vi "gugudan Client.vi"() -> ()   [LabVIEW 2014]
uses:
  <vilib>/Utility/sysdir.llb/System Directory Type.ctl
  <vilib>/regexp/Match Regular Expression.xnode
  <vilib>/FTP/NI_FTP.lvlib
panel:
  out "ip address":string=" ip address\r\n   서브넷 마스크 . . . . . . . : 255.255.255.0\r\n   기본 게이트웨이 . . . . . . : 192.168.0.1\r\n\r\n터널 어댑터 isatap.{E2E91750-802C-47E4-94E7-F6C5BD44A78B}:\r\n\r\n   미디어 상태 . . . . . . . . : 미디어 연결 끊김\r\n   연결별 DNS 접미사. . . . : \r\n\r\n터널 어댑터 로컬 영역 연결* 2:\r\n\r\n   연결별 DNS 접미사. . . . : \r\n   IPv6 주소 . . . . . . . . . : 2001:0:682f:9980:3c40:17a9:3f57:fff6\r\n   링크-로컬 IPv6 주소 . . . . : fe80::3c40:17a9:3f57:fff6%12\r\n   기본 게이트웨이 . . . . . . : ::\r\n"
  in  "제한해제":bool
  out "TIME":string="현재날자,시간"
  out "배열":string[][](array[string])
  out "email":string
  out "abs(x)":i32
  out "문자열":string
  out "스페이스바3 2":string
  out "W":string
  out "1":string
  out "2":string
  out "3":string
  # "서비스를 이용해 주셔 감사합니다."
  # "서비스 종료를 위해서는 관리자 암호를 입력 해야 종료가 가능합니다."
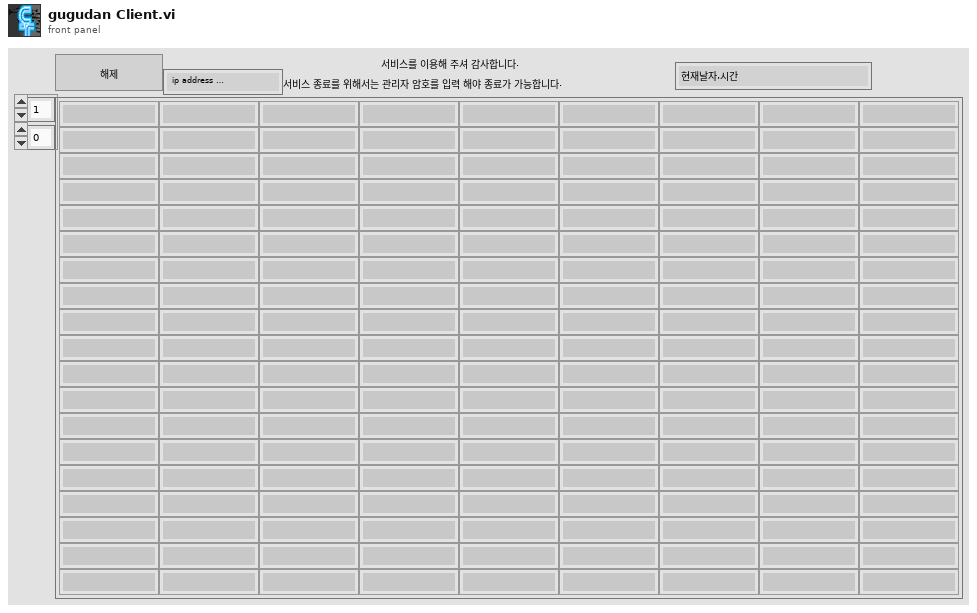
[diagram p1: front panel]
types:
  T1 = enum16{"open", "replace", "create", "open or create", "replace or create", "replace or create with confirmation"}
  T2 = typedef "System Directory Type.ctl" = i32
  T3 = typedef "NI_FTP.lvlib/FTP Session.ctl" = refnum<k5>
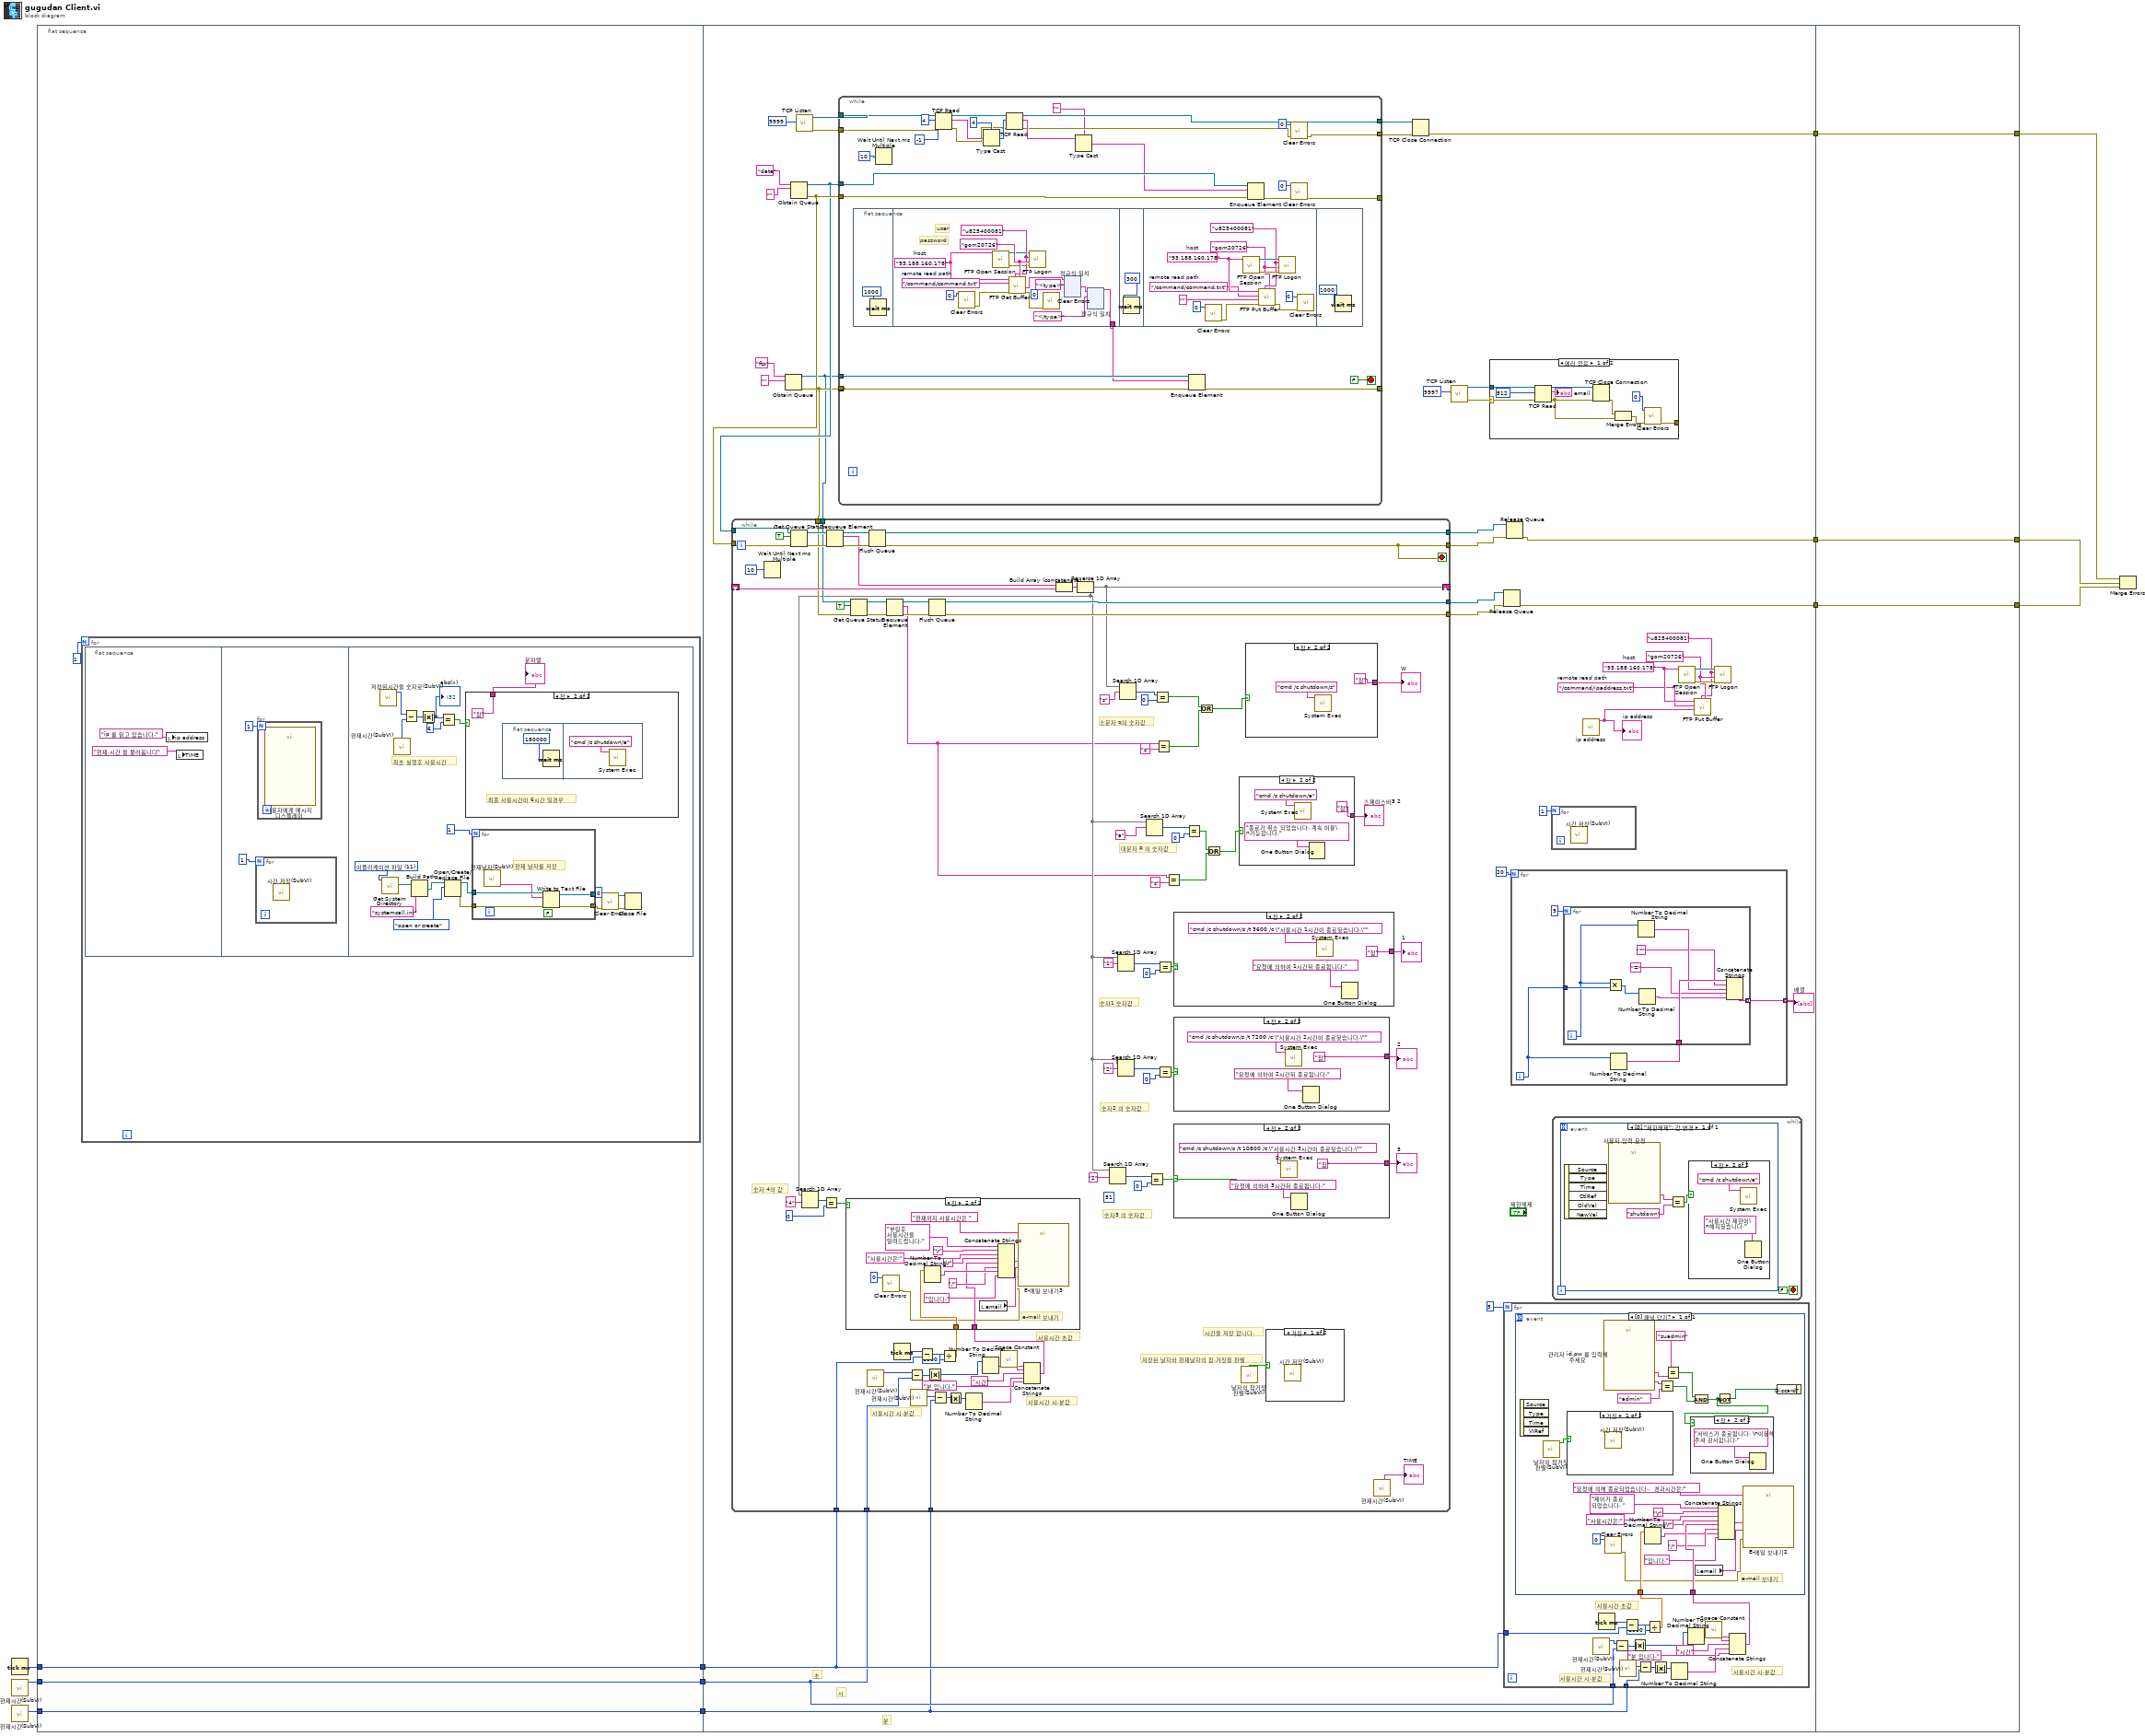
[diagram p0: block diagram]
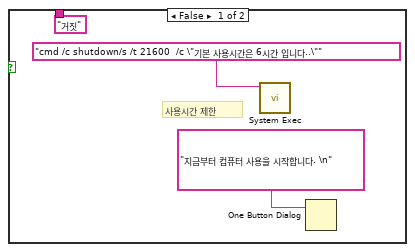
[diagram p2: hidden frame]
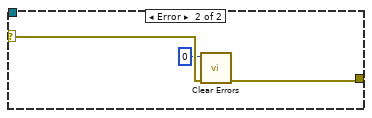
[diagram p4: hidden frame]
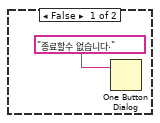
[diagram p6: hidden frame]
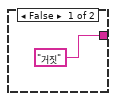
[diagram p9: hidden frame]
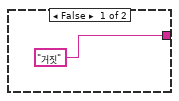
[diagram p10: hidden frame]
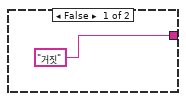
[diagram p11: hidden frame]
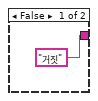
[diagram p12: hidden frame]
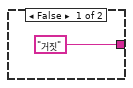
[diagram p13: hidden frame]
diagram:
  n1 = Tick Count (ms)() -> (millisecond timer value=w6:u32)
  n2 = call "현재시간(SubVI).vi"() -> ("시"=w5:i32)  [unwired: 3 in, 8 out]
  n3 = call "현재시간(SubVI).vi"() -> ("분"=w4:i32)  [unwired: 3 in, 8 out]
  n4 = flat-sequence {
    tunnel: [w15] -> w7
    tunnel: w6 -> [w15]
    tunnel: w5 -> [w14]
    tunnel: w4 -> [w13]
    tunnel: [w14] -> w3
    tunnel: [w13] -> w2
    tunnel: [w77] -> w12
    tunnel: [w73] -> w11
    tunnel: [w76] -> w10
    tunnel: w7 -> [w71]
    tunnel: w3 -> [w70]
    tunnel: w2 -> [w69]
    tunnel: w12 -> [w562]
    tunnel: w11 -> [w561]
    tunnel: w10 -> [w560]
    tunnel: [w562] -> w9
    tunnel: [w561] -> w8
    tunnel: [w560] -> w1
    frame #0 {
      n5 = for {
        N: 1 -> [_]
        n6 = flat-sequence {
          frame #0 {
            n7 = local write "ip address"("ip 를 읽고 있습니다.") -> ()
            n8 = local write "TIME"("현재,시간 을 불러옵니다") -> ()
          }
          frame #1 {
            n9 = for {
              N: 1 -> [_]
              n10 = call "시간 저장(SubVI).vi"() -> ()  [unwired: 12 in]
            }
            n11 = for {
              N: 1 -> [_]
              n12 = call "사용자에게 메시지 디스플레이"() -> ()  [unwired: 10 in, 2 out]
            }
          }
          frame #2 {
            w23 = T2 11 items=["사용자 홈"=0, "사용자 데스크탑"=1, "사용자 문서"=2, "사용자 어플리케이션 데이터"=3, "사용자 환경"=4, "사용자 임시"=5, "퍼블릭 문서"=6, "퍼블릭 어플리케이션 데이터"=7, "퍼블릭 환경"=8, "퍼블릭 캐시"=13, "시스템 코어 라이브러리"=9, "시스템 설치된 라이브러리"=10, "어플리케이션 파일"=11, "부팅 볼륨 루트"=12] ("system directory type")
            # "최초 실행후 사용시간"
            n13 = call "저장된시간을 숫자로(SubVI).vi"() -> ("저장된 문자를 숫자로"=w33:i32)  [unwired: 11 in]
            n14 = call <vilib>:"Get System Directory.vi"("system directory type"=w23) -> ("system directory"=w28:path)  [unwired: 10 in]
            n15 = call "현재시간(SubVI).vi"() -> ("시"=w34:i32)  [unwired: 3 in, 8 out]
            n16 = Subtract(x=w33, y=w34) -> (x-y=w35:i32)
            n17 = Build Path(base path=w28, name or relative path="systemcall.ini" ("이름 또는 상대 경로")) -> (appended path=w26:path)
            n18 = Absolute Value(x=w35) -> (abs(x)=w37:i32)
            "abs(x)" <- w37
            n19 = Equal?(x=w37, y=6) -> (x = y?=w39:bool)
            n20 = Open/Create/Replace File(file path (use dialog)=w26, operation (0:open)=T1."open or create" ("동작(0:open)")) -> (refnum out=w24:refnum<file>, error out=w25:errorcluster)  [unwired: 4 in, 1 out]
            n21 = case shown="참" w39 {
              tunnel: ["거짓" "참"] -> w36
              frame False {
                # "사용시간 제한"
                n22 = call <vilib>:"System Exec.vi"("command line"="cmd /c shutdown/s /t 21600  /c \"기본 사용시간은 6시간 입니다..\"" ("standard input")) -> ()  [unwired: 7 in, 4 out]
                n23 = One Button Dialog(message="지금부터 컴퓨터 사용을 시작합니다. \n" ("메시지")) -> ()  [unwired: 1 in, 1 out]
              }
              frame True {
                # "최종 사용시간이 6시간 일경우"
                n24 = flat-sequence {
                  frame #0 {
                    n25 = Wait (ms)(milliseconds to wait=u32 180000 ("대기 시간(ms)")) -> ()  [unwired: 1 out]
                  }
                  frame #1 {
                    n26 = call <vilib>:"System Exec.vi"("command line"="cmd /c shutdown/a" ("standard input")) -> ()  [unwired: 7 in, 4 out]
                  }
                }
              }
            }
            "문자열" <- w36
            n27 = for {
              N: 1 -> [_]
              tunnel: w25 -> [w44]
              tunnel: [w43] -> w30
              tunnel: [w42] -> w29
              tunnel: w24 -> [w41]
              (unwired) FALSE
              # "현재 날자를 저장"
              n28 = call "현재날자(SubVI).vi"() -> ("월,일 을 문자열로"=w40:string)  [unwired: 5 in, 6 out]
              n29 = Write to Text File(file (use dialog)=w41, text=w40, error in=w44) -> (refnum out=w42:refnum<file>, error out=w43:errorcluster)  [unwired: 1 in, 1 out]
            }
            n30 = call <vilib>:"Clear Errors.vi"("error in (no error)"=w30, "specific error code to clear (0: all)"=0) -> ("error out"=w31:errorcluster)  [unwired: 4 in, 1 out]
            n31 = Close File(refnum=w29, error in=w31) -> ()  [unwired: 2 out]
          }
        }
      }
    }
    frame #1 {
      w60 = "gom20726"
      w57 = "u825400081"
      w58 = "/command/ipaddress.txt"  # remote read path
      w59 = "93.188.160.178"  # host
      # "초"
      # "분"
      # "시"
      n32 = Obtain Queue(name (unnamed)="ftp" ("이름(이름없음)"), element data type="") -> (queue out=w52:refnum<queue>, error out=w53:errorcluster)  [unwired: 3 in, 1 out]
      n33 = Obtain Queue(name (unnamed)="data" ("이름(이름없음)"), element data type="") -> (queue out=w80:refnum<queue>, error out=w81:errorcluster)  [unwired: 3 in, 1 out]
      n34 = while {
        shift-right: [w175] -> _
        shift-left: _ -> [w227]
        tunnel: [w220] -> w83
        tunnel: [w219] -> w82
        tunnel: w80 -> [w226]
        tunnel: w81 -> [w225]
        tunnel: [w210] -> w79
        tunnel: [w209] -> w78
        tunnel: w52 -> [w205]
        tunnel: w53 -> [w204]
        tunnel: w71 -> [w185]
        tunnel: w70 -> [w184]
        tunnel: w69 -> [w183]
        stop <- w219 stop-if-true
        (unwired) i16 51 ("원소")
        # "숫자 4의 값"
        # "저장된 날자와 현재날자의 참,거짓을 판별"
        # "시간을 저장 합니다."
        # "사용시간 시,분값"
        # "사용시간 시,분값"
        # "사용시간 초값"
        # "대문자 R 의 숫자값"
        # "숫자3 의 숫자값"
        # "소문자 q의 숫자값"
        # "숫자1 숫자값"
        # "숫자2 의 숫자값"
        n35 = Wait Until Next ms Multiple(millisecond multiple=u32 10) -> ()  [unwired: 1 out]
        n36 = Get Queue Status(queue=w226, return elements? (F)=TRUE ("원소 반환? (거짓)"), error in (no error)=w225) -> (queue out=w224:refnum<queue>, error out=w223:errorcluster)  [unwired: 6 out]
        n37 = Dequeue Element(queue=w224, error in (no error)=w223) -> (queue out=w221:refnum<queue>, element=w218:string, error out=w222:errorcluster)  [unwired: 1 in, 1 out]
        n38 = Get Queue Status(queue=w205, return elements? (F)=TRUE ("원소 반환? (거짓)"), error in (no error)=w204) -> (queue out=w214:refnum<queue>, error out=w213:errorcluster)  [unwired: 6 out]
        n39 = call "현재시간(SubVI).vi"() -> ("시"=w187:i32)  [unwired: 3 in, 8 out]
        n40 = Flush Queue(queue=w221, error in (no error)=w222) -> (queue out=w220:refnum<queue>, error out=w219:errorcluster)  [unwired: 1 out]
        n41 = Dequeue Element(queue=w214, error in (no error)=w213) -> (queue out=w211:refnum<queue>, element=w167:string, error out=w212:errorcluster)  [unwired: 1 in, 1 out]
        n42 = Tick Count (ms)() -> (millisecond timer value=w186:u32)
        n43 = Subtract(x=w187, y=w184) -> (x-y=w189:i32)
        n44 = call "현재시간(SubVI).vi"() -> ("분"=w188:i32)  [unwired: 3 in, 8 out]
        n45 = Subtract(x=w186, y=w185) -> (x-y=w198:u32)
        n46 = Absolute Value(x=w189) -> (abs(x)=w191:i32)
        n47 = Flush Queue(queue=w211, error in (no error)=w212) -> (queue out=w209:refnum<queue>, error out=w210:errorcluster)  [unwired: 1 out]
        n48 = Subtract(x=w188, y=w183) -> (x-y=w190:i32)
        n49 = Divide(x=w198, y=u32 1000) -> (x/y=w182:dbl)
        n50 = Absolute Value(x=w190) -> (abs(x)=w192:i32)
        n51 = Number To Decimal String(number=w192) -> (decimal integer string=w194:string)  [unwired: 1 in]
        n52 = Number To Decimal String(number=w191) -> (decimal integer string=w196:string)  [unwired: 1 in]
        n53 = call <vilib>:"Space Constant.vi"() -> ("String"=w197:string)
        n54 = Concatenate Strings(w196, w197, "시간", w194, "분 입니다.") -> (w181:string)
        n55 = Build Array (concatenate)(w218, w227) -> (w216:string[])
        n56 = Reverse 1D Array(array=w216) -> (reversed array=w175:string[])
        n57 = Search 1D Array(1D array=w175, element="4") -> (index of element=w202:i32)  [unwired: 1 in]
        n58 = Equal?(x=w202, y=0) -> (x = y?=w200:bool)
        n59 = case shown="참" w200 {
          tunnel: w182 -> [_ w248]
          tunnel: w181 -> [_ w247]
          frame False {
          }
          frame True {
            # "e-mail 보내기"
            n60 = call <vilib>:"Clear Errors.vi"("specific error code to clear (0: all)"=0) -> ("error out"=w244:errorcluster)  [unwired: 5 in, 1 out]
            n61 = Number To Decimal String(number=w248) -> (decimal integer string=w256:string)  [unwired: 1 in]
            n62 = local read "email"() -> (w246:string)
            n63 = Concatenate Strings("부팅후 사용시간을 알려드립니다." ("문자열"), "\r", "사용시간은:", "\r", w247, "/", w256, "입니다.") -> (w253:string)
            n64 = call "E-메일 보내기3"("error in"=w244, "Message"=w253, "Subject"="현재까지 사용시간은 ", "Recipients"=w246) -> ()  [unwired: 7 in, 1 out]
          }
        }
        n65 = Search 1D Array(1D array=w175, element="2") -> (index of element=w232:i32)  [unwired: 1 in]
        n66 = Search 1D Array(1D array=w175, element="1" ("원소")) -> (index of element=w240:i32)  [unwired: 1 in]
        n67 = Search 1D Array(1D array=w175, element="2" ("원소")) -> (index of element=w233:i32)  [unwired: 1 in]
        n68 = Search 1D Array(1D array=w175, element="s" ("원소")) -> (index of element=w242:i32)  [unwired: 1 in]
        n69 = Search 1D Array(1D array=w175, element="a" ("원소")) -> (index of element=w207:i32)  [unwired: 1 in]
        n70 = Equal?(x=w232, y=0) -> (x = y?=w230:bool)
        n71 = Equal?(x=w242, y=0) -> (x = y?=w171:bool)
        n72 = Equal?(x=w167, y="s") -> (x = y?=w170:bool)
        n73 = Equal?(x=w240, y=0) -> (x = y?=w238:bool)
        n74 = Equal?(x=w233, y=0) -> (x = y?=w235:bool)
        n75 = Equal?(x=w167, y="s") -> (x = y?=w165:bool)
        n76 = case shown="참" w238 {
          tunnel: ["거짓" "참"] -> w239
          frame False {
          }
          frame True {
            n77 = call <vilib>:"System Exec.vi"("command line"="cmd /c shutdown/s /t 3600 /c \"사용시간 1시간이 종료됫습니다.\"" ("standard input")) -> ()  [unwired: 7 in, 4 out]
            n78 = One Button Dialog(message="요청에 의하여 1시간뒤 종료됩니다." ("메시지")) -> ()  [unwired: 1 in, 1 out]
          }
        }
        "1" <- w239
        n79 = case shown="참" w235 {
          tunnel: ["거짓" "참"] -> w234
          frame False {
          }
          frame True {
            n80 = call <vilib>:"System Exec.vi"("command line"="cmd /c shutdown/s /t 7200 /c \"사용시간 2시간이 종료됫습니다.\"" ("standard input")) -> ()  [unwired: 7 in, 4 out]
            n81 = One Button Dialog(message="요청에 의하여 2시간뒤 종료됩니다." ("메시지")) -> ()  [unwired: 1 in, 1 out]
          }
        }
        "2" <- w234
        n82 = case shown="참" w230 {
          tunnel: ["거짓" "참"] -> w217
          frame False {
          }
          frame True {
            n83 = call <vilib>:"System Exec.vi"("command line"="cmd /c shutdown/s /t 10800 /c \"사용시간 3시간이 종료됫습니다.\"" ("standard input")) -> ()  [unwired: 7 in, 4 out]
            n84 = One Button Dialog(message="요청에 의하여 3시간뒤 종료됩니다." ("메시지")) -> ()  [unwired: 1 in, 1 out]
          }
        }
        "3" <- w217
        n85 = Equal?(x=w207, y=0) -> (x = y?=w166:bool)
        n86 = Or(x=w171, y=w170) -> (x .or. y?=w169:bool)
        n87 = Or(x=w166, y=w165) -> (x .or. y?=w164:bool)
        n88 = case shown="참" w164 {
          tunnel: ["거짓" "참"] -> w206
          frame False {
          }
          frame True {
            n89 = call <vilib>:"System Exec.vi"("command line"="cmd /c shutdown/a" ("standard input")) -> ()  [unwired: 7 in, 4 out]
            n90 = One Button Dialog(message="종료가 취소 되었습니다. 계속 이용\n가능합니다." ("메시지")) -> ()  [unwired: 1 in, 1 out]
          }
        }
        "스페이스바3 2" <- w206
        n91 = call "날자의 참거짓 판별(SubVI).vi"() -> ("불리언"=w203:bool)  [unwired: 9 in, 2 out]
        n92 = case shown="참" w169 {
          tunnel: ["거짓" "참"] -> w243
          frame False {
          }
          frame True {
            n93 = call <vilib>:"System Exec.vi"("command line"="cmd /c shutdown/s" ("standard input")) -> ()  [unwired: 7 in, 4 out]
          }
        }
        "W" <- w243
        n94 = case shown="거짓" w203 {
          frame False {
            n95 = call "시간 저장(SubVI).vi"() -> ()  [unwired: 12 in]
          }
          frame True {
          }
        }
        n96 = call "현재시간(SubVI).vi"() -> ("날짜/시간 문자열"=→"TIME":string)  [unwired: 3 in, 8 out]
      }
      n97 = call <vilib>:"TCP Listen.vi"("port"=u16 9999) -> ("error out"=w74:errorcluster, "connection ID"=w85:refnum<k5>)  [unwired: 6 in, 3 out]
      n98 = while {
        tunnel: w85 -> [w283]
        tunnel: [w303] -> w86
        tunnel: w80 -> [w296]
        tunnel: w81 -> [w295]
        tunnel: [w289] -> w75
        tunnel: w74 -> [w290]
        tunnel: [w286] -> _
        tunnel: w52 -> [w281]
        tunnel: [w280] -> _
        tunnel: w53 -> [w280]
        tunnel: [w279] -> _
        stop <- FALSE stop-if-true
        n99 = flat-sequence {
          tunnel: [w305] -> w278
          frame #0 {
            n100 = Wait (ms)(milliseconds to wait=u32 1000 ("대기 시간(ms)")) -> ()  [unwired: 1 out]
          }
          frame #1 {
            (unwired) 0 ("specific error code to clear (0: all)")
            w309 = "gom20726"
            w308 = "u825400081"
            w311 = "/command/command.txt"  # remote read path
            w310 = "93.188.160.178"  # host
            # "user"
            # "password"
            n101 = call <vilib>:"Clear Errors.vi"("specific error code to clear (0: all)"=0) -> ("error out"=w312:errorcluster)  [unwired: 5 in, 1 out]
            n102 = call <vilib>:"FTP Open Session.vi"("address"=w310) -> ("error out"=w307:errorcluster, "ftp session"=w306:T3)  [unwired: 7 in, 2 out]
            n103 = call <vilib>:"FTP Get Buffer.vi"("password"=w309, "user"=w308, "error in (no error)"=w312, "remote path"=w311, "host"=w310) -> ("error out"=w314:errorcluster, "data"=w315:string)  [unwired: 4 in, 1 out]
            n104 = call <vilib>:"FTP Logon.vi"("error in (no error)"=w307, "password"=w309, "user"=w308, "ftp session"=w306) -> ()  [unwired: 4 in, 4 out]
            n105 = call <vilib>:"Clear Errors.vi"("error in (no error)"=w314) -> ()  [unwired: 5 in, 2 out]
            n106 = xnode "정규식 일치"("입력 문자열"=w315, "정규식"="<type>") -> ("일치 구문 뒤"=w317:string)  [unwired: 4 in, 4 out]
            n107 = xnode "정규식 일치"("입력 문자열"=w317, "정규식"="</type>") -> ("일치 구문 앞"=w305:string)  [unwired: 4 in, 4 out]
          }
          frame #2 {
            n108 = Wait (ms)(milliseconds to wait=u32 300 ("대기 시간(ms)")) -> ()  [unwired: 1 out]
          }
          frame #3 {
            w555 = "gom20726"
            w556 = "u825400081"
            w553 = "/command/command.txt"  # remote read path
            w554 = "93.188.160.178"  # host
            n109 = call <vilib>:"Clear Errors.vi"("specific error code to clear (0: all)"=0) -> ("error out"=w551:errorcluster)  [unwired: 5 in, 1 out]
            n110 = call <vilib>:"FTP Open Session.vi"("address"=w554) -> ("error out"=w557:errorcluster, "ftp session"=w558:T3)  [unwired: 7 in, 2 out]
            n111 = call <vilib>:"FTP Put Buffer.vi"("password"=w555, "user"=w556, "error in (no error)"=w551, "data"="", "remote path"=w553, "host"=w554) -> ("error out"=w549:errorcluster)  [unwired: 4 in, 1 out]
            n112 = call <vilib>:"FTP Logon.vi"("error in (no error)"=w557, "password"=w555, "user"=w556, "ftp session"=w558) -> ()  [unwired: 4 in, 4 out]
            n113 = call <vilib>:"Clear Errors.vi"("error in (no error)"=w549, "specific error code to clear (0: all)"=0) -> ()  [unwired: 4 in, 2 out]
          }
          frame #4 {
            n114 = Wait (ms)(milliseconds to wait=u32 1000 ("대기 시간(ms)")) -> ()  [unwired: 1 out]
          }
        }
        n115 = Wait Until Next ms Multiple(millisecond multiple=u32 10) -> ()  [unwired: 1 out]
        n116 = TCP Read(connection ID=w283, bytes to read=4, error in (no error)=w290, 9:-1 ("타임아웃 ms (25000)")) -> (connection ID out=w299:refnum<k5>, data out=w301:string, error out=w291:errorcluster)  [unwired: 1 in]
        n117 = Type Cast(type=4 ("bytes to read"), x=w301) -> (*(type *) &x=w293:i32)
        n118 = TCP Read(connection ID=w299, bytes to read=w293, error in (no error)=w291) -> (connection ID out=w303:refnum<k5>, data out=w294:string, error out=w288:errorcluster)  [unwired: 2 in]
        n119 = Type Cast(type="", x=w294) -> (*(type *) &x=w277:string)
        n120 = Enqueue Element(queue=w281, element=w278, error in (no error)=w280) -> (error out=w279:errorcluster)  [unwired: 1 in, 2 out]
        n121 = Enqueue Element(queue=w296, element=w277, error in (no error)=w295) -> (error out=w287:errorcluster)  [unwired: 1 in, 2 out]
        n122 = call <vilib>:"Clear Errors.vi"("error in (no error)"=w288, "specific error code to clear (0: all)"=0) -> ("error out"=w289:errorcluster)  [unwired: 4 in, 1 out]
        n123 = call <vilib>:"Clear Errors.vi"("error in (no error)"=w287, "specific error code to clear (0: all)"=0) -> ("error out"=w286:errorcluster)  [unwired: 4 in, 1 out]
      }
      n124 = TCP Close Connection(connection ID=w86, error in (no error)=w75) -> (error out=w76:errorcluster)  [unwired: 1 in, 1 out]
      n125 = call <vilib>:"TCP Listen.vi"("port"=u16 9997) -> ("error out"=w66:errorcluster, "connection ID"=w67:refnum<k5>)  [unwired: 6 in, 3 out]
      n126 = case shown="에러 없음" w66 {
        selector: w66 -> [w112 w118]
        tunnel: [w109 w119] -> _
        tunnel: w67 -> [w116 _]
        frame No Error {
          n127 = TCP Read(connection ID=w116, bytes to read=512, error in (no error)=w112) -> (connection ID out=w111:refnum<k5>, data out=→"email":string, error out=w110:errorcluster)  [unwired: 2 out]
          n128 = TCP Close Connection(connection ID=w111, error in (no error)=w110) -> (error out=w113:errorcluster)  [unwired: 2 out]
          n129 = Merge Errors(w113, w110) -> (w108:errorcluster)
          n130 = call <vilib>:"Clear Errors.vi"("error in (no error)"=w108, "specific error code to clear (0: all)"=0) -> ("error out"=w109:errorcluster)  [unwired: 4 in, 1 out]
        }
        frame Error {
          n131 = call <vilib>:"Clear Errors.vi"("error in (no error)"=w118, "specific error code to clear (0: all)"=0) -> ("error out"=w119:errorcluster)  [unwired: 4 in, 1 out]
        }
      }
      n132 = Release Queue(queue=w78, error in (no error)=w79) -> (error out=w73:errorcluster)  [unwired: 1 in, 2 out]
      n133 = for {
        N: 5 -> [_]
        tunnel: w71 -> [w137]
        tunnel: w70 -> [w135]
        tunnel: w69 -> [w133]
        # "사용시간 시,분값"
        # "사용시간 시,분값"
        # "사용시간 초값"
        n134 = call "현재시간(SubVI).vi"() -> ("시"=w136:i32)  [unwired: 3 in, 8 out]
        n135 = Tick Count (ms)() -> (millisecond timer value=w138:u32)
        n136 = Subtract(x=w136, y=w135) -> (x-y=w132:i32)
        n137 = call "현재시간(SubVI).vi"() -> ("분"=w134:i32)  [unwired: 3 in, 8 out]
        n138 = Subtract(x=w138, y=w137) -> (x-y=w123:u32)
        n139 = Absolute Value(x=w132) -> (abs(x)=w130:i32)
        n140 = Subtract(x=w134, y=w133) -> (x-y=w131:i32)
        n141 = Divide(x=w123, y=u32 1000) -> (x/y=w121:dbl)
        n142 = Absolute Value(x=w131) -> (abs(x)=w129:i32)
        n143 = Number To Decimal String(number=w129) -> (decimal integer string=w127:string)  [unwired: 1 in]
        n144 = Number To Decimal String(number=w130) -> (decimal integer string=w125:string)  [unwired: 1 in]
        n145 = call <vilib>:"Space Constant.vi"() -> ("String"=w124:string)
        n146 = Concatenate Strings(w125, w124, "시간", w127, "분 입니다.") -> (w120:string)
        n147 = event shown="[0] 패널 닫기?" {
          selector: _ -> [_]
          dyn-events: _ -> [_]
          timeout: _ -> [_]
          tunnel: w121 -> [w153]
          tunnel: w120 -> [w146]
          event Panel Close? {
            # "e-mail 보내기"
            n148 = event-data() -> ()  [unwired: 1 in, 4 out]
            n149 = call "날자의 참거짓 판별(SubVI).vi"() -> ("불리언"=w142:bool)  [unwired: 9 in, 2 out]
            n150 = case shown="거짓" w142 {
              frame False {
                n151 = call "시간 저장(SubVI).vi"() -> ()  [unwired: 12 in]
              }
              frame True {
              }
            }
            n152 = call "관리자 id.pw 를 입력해 주세요"() -> ("PW"=w161:string, "ID"=w158:string)  [unwired: 16 in, 2 out]
            n153 = call <vilib>:"Clear Errors.vi"("specific error code to clear (0: all)"=0) -> ("error out"=w140:errorcluster)  [unwired: 5 in, 1 out]
            n154 = Number To Decimal String(number=w153) -> (decimal integer string=w144:string)  [unwired: 1 in]
            n155 = Equal?(x=w161, y="admin") -> (x = y?=w157:bool)
            n156 = Equal?(x="suadmin", y=w158) -> (x = y?=w156:bool)
            n157 = And(x=w156, y=w157) -> (x .and. y?=w154:bool)
            n158 = case shown="참" w154 {
              frame False {
                n159 = One Button Dialog(message="종료할수 없습니다." ("메시지")) -> ()  [unwired: 1 in, 1 out]
              }
              frame True {
                n160 = One Button Dialog(message="서비스가 종료됩니다. \n이용해 주셔 감사합니다." ("메시지")) -> ()  [unwired: 1 in, 1 out]
              }
            }
            n161 = local read "email"() -> (w141:string)
            n162 = Not(x=w154) -> (.not. x?=w155:bool)
            n163 = Concatenate Strings("제어가 종료 되었습니다. " ("문자열"), "\r", "사용시간은:", "\r", w146, "/", w144, "입니다.") -> (w148:string)
            n164 = call "E-메일 보내기2"("error in"=w140, "Message"=w148, "Subject"="요청에 의해 종료되었습니다,.  경과시간은:", "Recipients"=w141) -> ()  [unwired: 7 in, 1 out]
            n165 = event-data("Discard?"=w155) -> ()  [unwired: 1 in, 1 out]
          }
        }
      }
      n166 = Release Queue(queue=w83, error in (no error)=w82) -> (error out=w77:errorcluster)  [unwired: 1 in, 2 out]
      n167 = for {
        N: 20 -> [_]
        tunnel: [w94] -> w64 mode=indexing
        i -> [w96]
        n168 = Number To Decimal String(number=w96) -> (decimal integer string=w95:string)  [unwired: 1 in]
        n169 = for {
          N: 9 -> [_]
          tunnel: w96 -> [w106]
          tunnel: w95 -> [w104]
          tunnel: [w99] -> w94 mode=indexing
          i -> [w98]
          n170 = Multiply(x=w98, y=w106) -> (x*y=w105:i32)
          n171 = Number To Decimal String(number=w98) -> (decimal integer string=w103:string)  [unwired: 1 in]
          n172 = Number To Decimal String(number=w105) -> (decimal integer string=w100:string)  [unwired: 1 in]
          n173 = Concatenate Strings(w104, "*", w103, "=", w100) -> (w99:string)
        }
      }
      "배열" <- w64
      n174 = for {
        N: 1 -> [_]
        n175 = call "시간 저장(SubVI).vi"() -> ()  [unwired: 12 in]
      }
      n176 = while {
        stop <- FALSE stop-if-true
        n177 = event shown="[0] \"제한해제\": 값 변경" {
          selector: _ -> [_]
          dyn-events: _ -> [_]
          timeout: _ -> [_]
          event "제한해제": Value Change {
            n178 = event-data() -> ()  [unwired: 1 in, 6 out]
            n179 = call "사용자 입력 요청"() -> ("종료 취소"=w90:string)  [unwired: 17 in, 2 out]
            n180 = Equal?(x=w90, y="shutdown") -> (x = y?=w89:bool)
            n181 = case shown="참" w89 {
              frame False {
              }
              frame True {
                n182 = call <vilib>:"System Exec.vi"("command line"="cmd /c shutdown/a" ("standard input")) -> ()  [unwired: 7 in, 4 out]
                n183 = One Button Dialog(message="사용시간 제한이\n해지됫습니다." ("메시지")) -> ()  [unwired: 1 in, 1 out]
              }
            }
          }
        }
      }
      n184 = call "ip address.vi"() -> ("ip address"=w56:string)  [unwired: 11 in]
      "ip address" <- w56
      n185 = call <vilib>:"FTP Open Session.vi"("address"=w59) -> ("error out"=w61:errorcluster, "ftp session"=w62:T3)  [unwired: 7 in, 2 out]
      n186 = call <vilib>:"FTP Put Buffer.vi"("password"=w60, "user"=w57, "data"=w56, "remote path"=w58, "host"=w59) -> ()  [unwired: 5 in, 2 out]
      n187 = call <vilib>:"FTP Logon.vi"("error in (no error)"=w61, "password"=w60, "user"=w57, "ftp session"=w62) -> ()  [unwired: 4 in, 4 out]
    }
    frame #2 {
    }
  }
  n188 = Merge Errors(w1, w9, w8) -> ()  [unwired: 1 out]
